vi "Scan.vi"(3 "SN":string caption="SN: Length should be 12") -> ()   [LabVIEW 2013]
uses:
  Global constant.vi
panel:
  in  "OK Button":bool
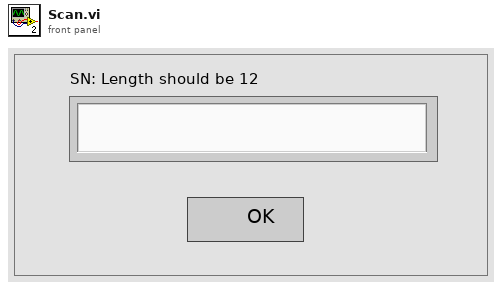
[diagram p1: front panel]
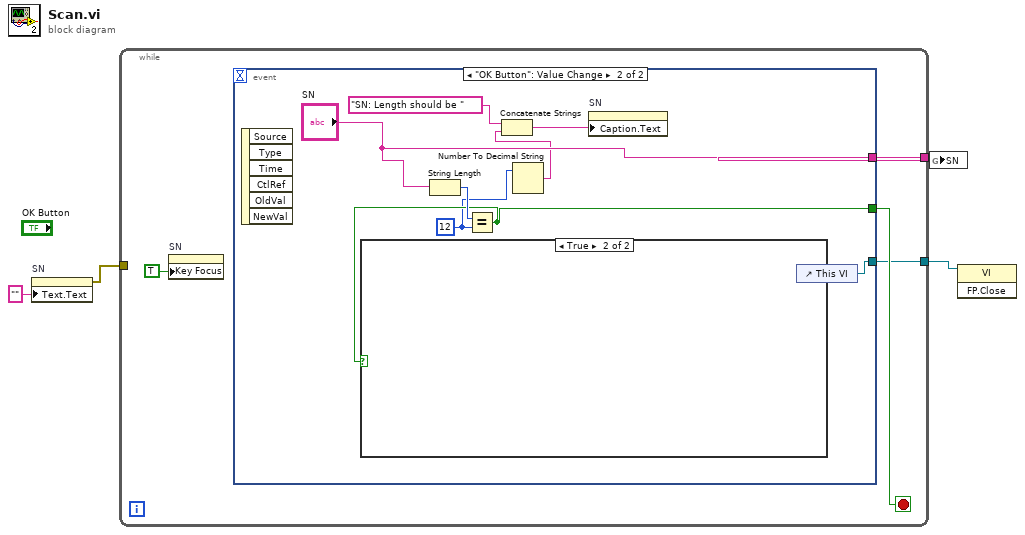
[diagram p0: block diagram]
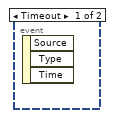
[diagram p2: hidden frame]
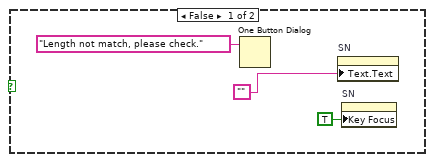
[diagram p3: hidden frame]
diagram:
  n1 = property on="SN" class="Str"("Text.Text"="") -> (error out=w1:errorcluster)  [unwired: 2 in, 1 out]
  n2 = while {
    tunnel: [w6] -> w3
    tunnel: [w5] -> w2
    tunnel: w1 -> [_]
    stop <- w8 stop-if-true
    n3 = property on="SN" class="Str"("Key Focus"=TRUE) -> ()  [unwired: 2 in, 2 out]
    n4 = event shown="[1] \"OK Button\": Value Change" {
      selector: _ -> [_ _]
      dyn-events: _ -> [_ _]
      timeout: _ -> [_ _]
      tunnel: [_ w13] -> w8
      tunnel: [_ "SN"] -> w6
      tunnel: [_ w15] -> w5
      event Timeout {
        n5 = event-data() -> ()  [unwired: 1 in, 3 out]
      }
      event "OK Button": Value Change {
        w10 = 12 ("y")
        n6 = event-data() -> ()  [unwired: 1 in, 6 out]
        n7 = String Length(string="SN") -> (length=w16:i32)
        n8 = Equal?(x=w16, y=w10) -> (x = y?=w13:bool)
        n9 = case shown="True" w13 {
          frame False {
            n10 = One Button Dialog(message="Length not match, please check.") -> ()  [unwired: 1 in, 1 out]
            n11 = property on="SN" class="Str"("Text.Text"="") -> ()  [unwired: 2 in, 2 out]
            n12 = property on="SN" class="Str"("Key Focus"=TRUE) -> ()  [unwired: 2 in, 2 out]
          }
          frame True {
          }
        }
        n13 = Number To Decimal String(number=w10) -> (decimal integer string=w9:string)  [unwired: 1 in]
        n14 = Concatenate Strings("SN: Length should be " ("string"), w9) -> (w11:string)
        n15 = property on="SN" class="Str"("Caption.Text"=w11) -> ()  [unwired: 2 in, 2 out]
        n16 = control-ref of="This VI"() -> (w15:refnum<vi>)
      }
    }
  }
  n17 = global write "Global constant.vi" "SN"(w3) -> ()
  n18 = invoke class="VI" method="FP.Close"(reference=w2) -> ()  [unwired: 2 in, 3 out]
